vi "Keithley 2002 Set Output.vi"(1 "ch4 level":bool, 2 "ch3 level":bool, 3 "ch2 level":bool, 4 "ch1 level":bool, 5 "ch4 polarity":bool=TRUE, 6 "ch3 polarity":bool=TRUE, 7 "error in":T1, 8 "ch2 polarity":bool=TRUE, 9 "ch1 polarity":bool=TRUE, 10 "GPIB address":string="16") -> (0 "error out":T1)   [LabVIEW 2020]
doc: "This VI is used to control the 4 digital output lines of the instrument. The polarity can be set to active-high or active-low and the channels can be turned on or off on an individual basis."
panel:
  # "high\nlow"
  # "on\noff"
  # "high\nlow"
  # "on\noff"
  # "high\nlow"
  # "on\noff"
  # "high\nlow"
  # "on\noff"
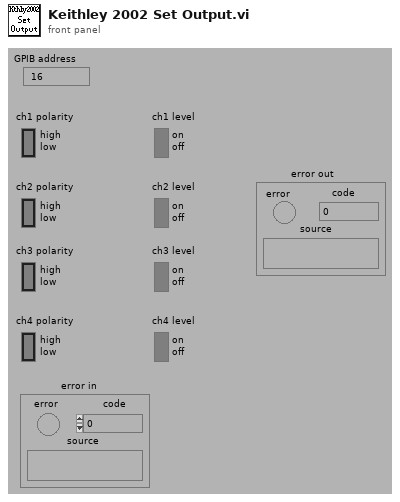
[diagram p1: front panel]
types:
  T1 = cluster{"error":bool, "code":i32, "source":string}
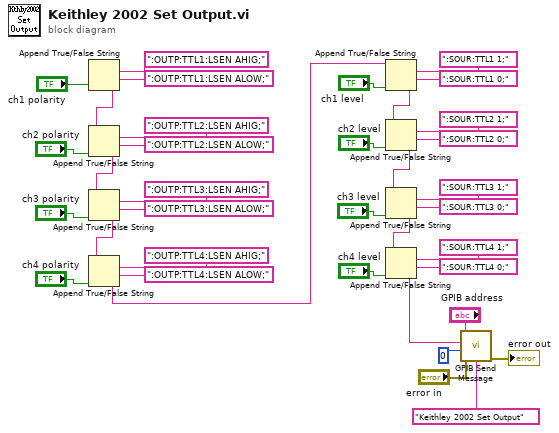
[diagram p0: block diagram]
diagram:
  n1 = Append True/False String(1:"ch1 polarity", 2:":OUTP:TTL1:LSEN ALOW;", 3:":OUTP:TTL1:LSEN AHIG;") -> (0:w28:string)  [unwired: 1 in]
  n2 = Append True/False String(1:"ch2 polarity", 2:":OUTP:TTL2:LSEN ALOW;", 3:":OUTP:TTL2:LSEN AHIG;", 4:w28) -> (0:w18:string)
  n3 = Append True/False String(1:"ch3 polarity", 2:":OUTP:TTL3:LSEN ALOW;", 3:":OUTP:TTL3:LSEN AHIG;", 4:w18) -> (0:w25:string)
  n4 = Append True/False String(1:"ch4 polarity", 2:":OUTP:TTL4:LSEN ALOW;", 3:":OUTP:TTL4:LSEN AHIG;", 4:w25) -> (0:w16:string)
  n5 = Append True/False String(1:"ch1 level", 2:":SOUR:TTL1 0;", 3:":SOUR:TTL1 1;", 4:w16) -> (0:w9:string)
  n6 = Append True/False String(1:"ch2 level", 2:":SOUR:TTL2 0;", 3:":SOUR:TTL2 1;", 4:w9) -> (0:w8:string)
  n7 = Append True/False String(1:"ch3 level", 2:":SOUR:TTL3 0;", 3:":SOUR:TTL3 1;", 4:w8) -> (0:w7:string)
  n8 = Append True/False String(1:"ch4 level", 2:":SOUR:TTL4 0;", 3:":SOUR:TTL4 1;", 4:w7) -> (0:w1:string)
  n9 = call "GPIB Send Message.vi"("address string"="GPIB address", "write buffer"=w1, "source"="Keithley 2002 Set Output", "write mode (set END:0)"=0, "error in"="error in") -> ("error out"=→"error out":T1)  [unwired: 2 in, 2 out]
